vi "Number of Results in Case.vi"() -> (3 "Number of Results":i32)   [LabVIEW 2020, in "Test Case Test Double.lvclass"]
uses:
  Test Case Test Double.lvclass
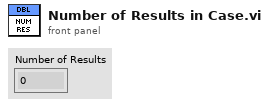
[diagram p1: front panel]
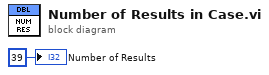
[diagram p0: block diagram]
diagram:
  "Number of Results" <- 39 ("Number of tests")
